vi "VIPM_Remove Path Duplicates.vi"(11 "Package Array in":T1[](array[typedef])) -> (3 "Package Array out":T1[](array[typedef]))   [LabVIEW 2019, in "Project.Dependencies Finder.lvlib" / "Dependency Source_VIPM.lvclass"]
doc: "Remove paths that are found more than once as these are non unique and cannot be used as identifiers."
uses:
  Dependency Source_VIPM.lvclass
  Ctl/Ctl_Package Identifier Cluster.ctl
  Project.Dependencies Finder.lvlib
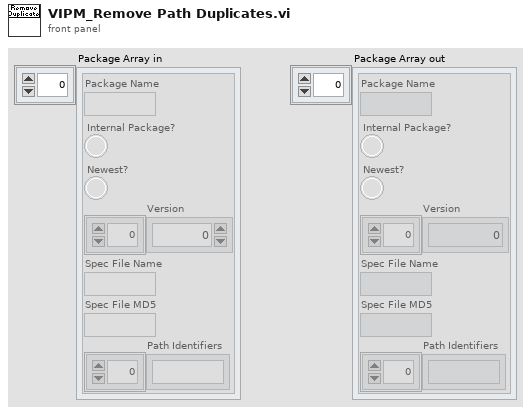
[diagram p1: front panel]
types:
  T1 = typedef "Project.Dependencies Finder.lvlib/Dependency Source_VIPM.lvclass/Ctl_Package Identifier Cluster.ctl" = cluster{"Package Name":string, "Internal Package?":bool, "Newest?":bool, "Version":i32[], "Spec File Name":string, "Spec File MD5":string, "Path Identifiers":string[]}
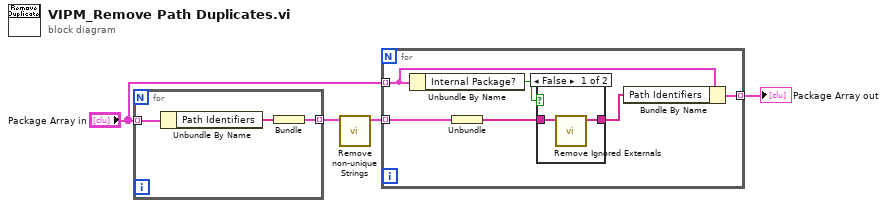
[diagram p0: block diagram]
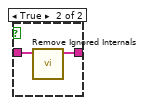
[diagram p2: hidden frame]
diagram:
  n1 = for {
    tunnel: "Package Array in" -> [w7] mode=indexing
    tunnel: [w5] -> w4 mode=indexing
    n2 = Unbundle By Name(w7) -> ("Path Identifiers"=w6:string[])
    n3 = Bundle("Path Identifiers"=w6) -> (w5:cluster{"Path Identifiers":string[]})  [unwired: 1 in]
  }
  n4 = call "Remove non-unique Strings.vi"("String Array in"=w4) -> ("String Array out"=w2:cluster{"Array":string[]}[])  [unwired: 9 in, 1 out]
  n5 = for {
    tunnel: "Package Array in" -> [w11] mode=indexing
    tunnel: w2 -> [w13] mode=indexing
    tunnel: [w12] -> w1 mode=indexing
    n6 = Unbundle By Name(w11) -> ("Internal Package?"=w10:bool)
    n7 = Unbundle(w13) -> ("Array"=w9:string[])
    n8 = case shown="False" w10 {
      tunnel: w9 -> [w15 w17]
      tunnel: [w14 w16] -> w8
      frame False {
        n9 = call "Remove Ignored Externals.vi"("Externals in"=w15) -> ("Externals out"=w14:string[])  [unwired: 10 in]
      }
      frame True {
        n10 = call "Remove Ignored Internals.vi"("Internals in"=w17) -> ("Internals out"=w16:string[])  [unwired: 10 in]
      }
    }
    n11 = Bundle By Name(cluster=w11, "Path Identifiers"=w8) -> (w12:T1)
  }
  "Package Array out" <- w1
